vi "Insert Rows At (String).vi"(7 "image path":path, 8 "error in (no error)":errorcluster, 9 "String Data":string[][](array[string]), 10 "index":i32, 11 "DataTable in":refnum<class "DataTable.lvclass">) -> (0 "error out":errorcluster, 3 "DataTable out":refnum<class "DataTable.lvclass">)   [LabVIEW 2016, in "DataGrid.lvlib" / "DataTable.lvclass"]
doc: "This allows any number of rows to be added to the datatable. The data must match the columns defined for the grid."
uses:
  <userlib>/LabVIEWdotNetDataGrid/source/DataTable/DataTable.lvclass
  <userlib>/LabVIEWdotNetDataGrid/source/DataTable/DataTable.lvclass/DataTable.ctl
  System.Data
  <userlib>/LabVIEWdotNetDataGrid/source/GridColumn/GridColumn.lvclass/GridColumn.ctl
  <userlib>/LabVIEWdotNetDataGrid/source/GridColumn/Read datatype.vi
  <userlib>/LabVIEWdotNetDataGrid/source/GridColumn/GridColumn.lvclass
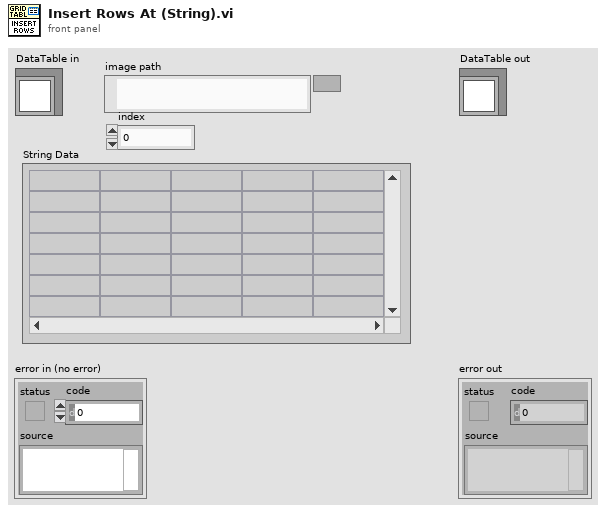
[diagram p1: front panel]
types:
  T1 = typedef "DataGrid.lvlib/GridColumn.lvclass/ColumnType.ctl" = enum16{"string", "image", "check", "numeric", "timestamp", "button", "combo", "link"}
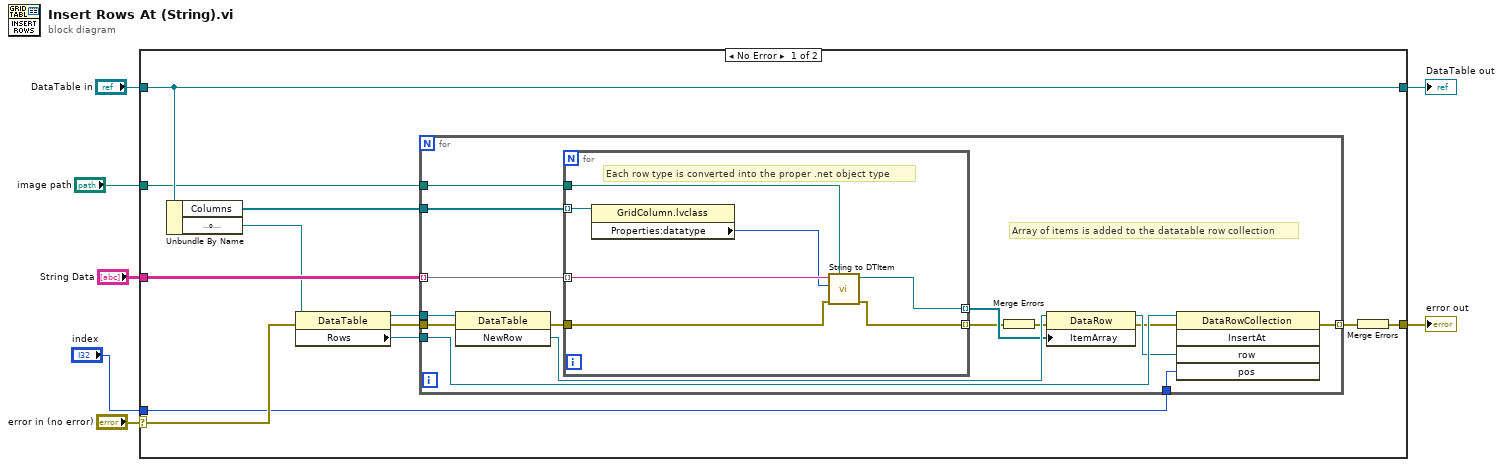
[diagram p0: block diagram]
diagram:
  n1 = case shown="No Error" "error in (no error)" {
    selector: "error in (no error)" -> [w16 w42]
    tunnel: [w17 w43] -> w5
    tunnel: "DataTable in" -> [w17 w43]
    tunnel: "String Data" -> [w15 _]
    tunnel: [w12 w42] -> w3
    tunnel: "image path" -> [w10 _]
    tunnel: "index" -> [w9 _]
    frame No Error {
      n2 = Unbundle By Name(w17) -> ("Columns"=w11:refnum<class "GridColumn.lvclass">[], "DataTable"=w14:refnum<k24>)
      n3 = property class="DataTable"(reference=w14, error in=w16) -> (reference out=w13:refnum<k24>, error out=w8:errorcluster, "Rows"=w19:refnum<k24>)
      n4 = for {
        tunnel: w19 -> [w33]
        tunnel: w13 -> [w34]
        tunnel: [w20] -> w18 mode=indexing
        tunnel: w15 -> [w32] mode=indexing
        tunnel: w8 -> [w26]
        tunnel: w11 -> [w25]
        tunnel: w10 -> [w24]
        tunnel: w9 -> [w23]
        # "Array of items is added to the datatable row collection"
        n5 = invoke class="DataTable" method="NewRow"(reference=w34, error in=w26) -> (error out=w31:errorcluster, "NewRow"=w30:refnum<k24>)  [unwired: 1 in, 1 out]
        n6 = for {
          tunnel: w32 -> [w39] mode=indexing
          tunnel: [w35] -> w28 mode=indexing
          tunnel: w31 -> [w37]
          tunnel: [w36] -> w27 mode=indexing
          tunnel: w25 -> [w41] mode=indexing
          tunnel: w24 -> [w40]
          # "Each row type is converted into the proper .net object type"
          n7 = property class="GridColumn.lvclass"(reference=w41) -> ("Properties:datatype"=w38:T1)  [unwired: 1 in, 2 out]
          n8 = call <userlib>:"String to DTItem.vi"("image path"=w40, "error in (no error)"=w37, "datatype"=w38, "element"=w39) -> ("error out"=w36:errorcluster, "DTItem .NET Refnum out"=w35:refnum<k24>)  [unwired: 6 in]
        }
        n9 = Merge Errors(w27) -> (w22:errorcluster)
        n10 = property class="DataRow"(reference=w30, error in=w22, "ItemArray"=w28) -> (reference out=w29:refnum<k24>, error out=w21:errorcluster)
        n11 = invoke class="DataRowCollection" method="InsertAt"(reference=w33, error in=w21, "row"=w29, "pos"=w23) -> (error out=w20:errorcluster)  [unwired: 1 in, 4 out]
      }
      n12 = Merge Errors(w18) -> (w12:errorcluster)
    }
    frame Error {
    }
  }
  "error out" <- w3
  "DataTable out" <- w5
